vi "Untitled 1.vi"() -> ()   [LabVIEW 2015]
panel:
  in  "length":i32
  in  "x":dbl(slide) scale=0.0..10.0
  in  "y":dbl(slide) scale=0.0..10.0
  out "XY Graph":cluster{"x":dbl, "y":dbl}[](graph)
  in  "nr punktu do usuniêcia":dbl
  in  "usuñ punkt o numerze":bool
  in  "usuñ ostatni punkt":bool
  in  "rysuj punkt":bool
  in  "stop":bool
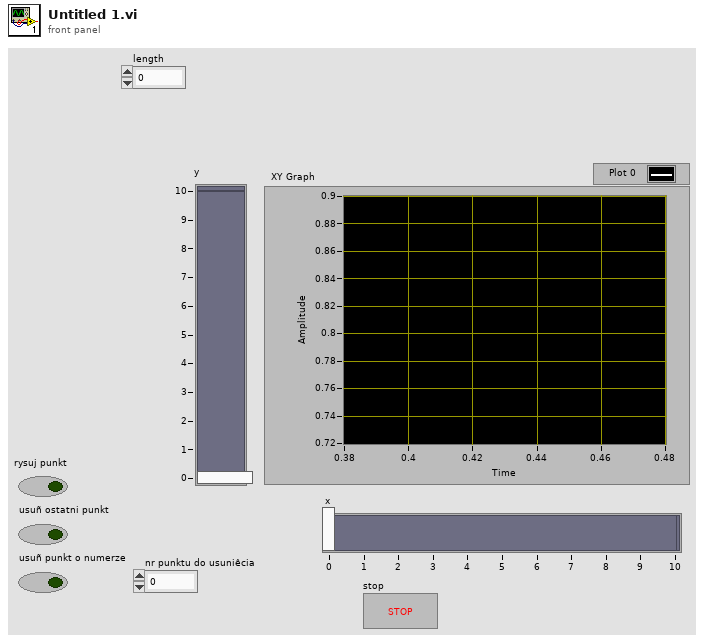
[diagram p1: front panel]
types:
  T1 = typedef "LVPoint32TypeDef.ctl" = cluster{"Horizontal":i32, "Vertical":i32}
  T2 = typedef "LVRectTypeDef.ctl" = cluster{"Left":i16, "Top":i16, "Right":i16, "Bottom":i16}
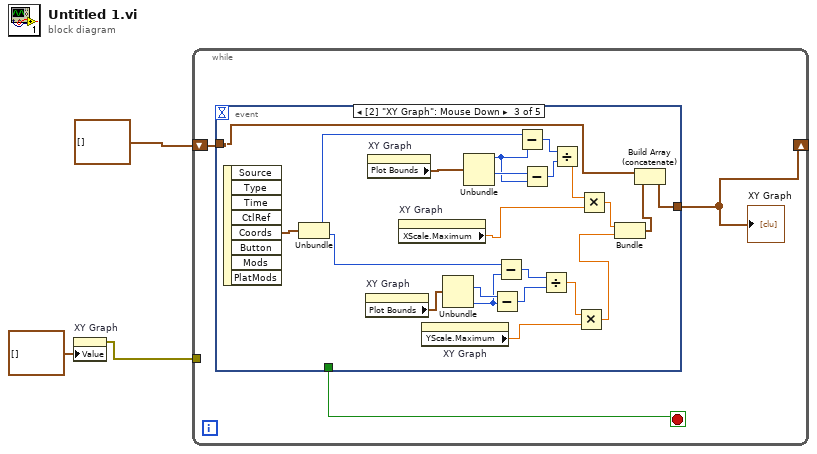
[diagram p0: block diagram]
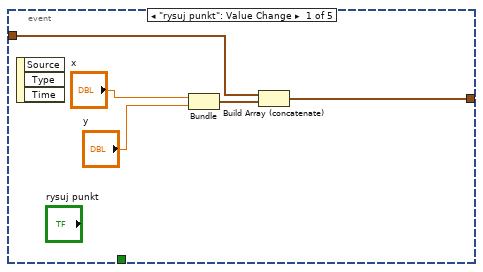
[diagram p2: hidden frame]
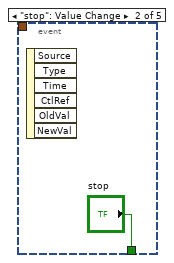
[diagram p3: hidden frame]
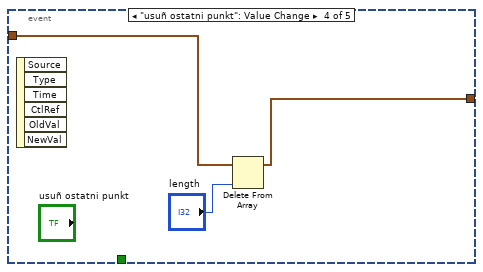
[diagram p4: hidden frame]
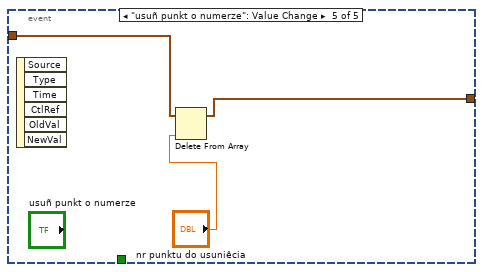
[diagram p5: hidden frame]
diagram:
  n1 = property on="XY Graph" class="XYGraph (strict)"("Value"=cluster{"x":dbl, "y":dbl}[] [] ("XY Graph")) -> (error out=w3:errorcluster)  [unwired: 2 in, 1 out]
  n2 = while {
    tunnel: w3 -> [_]
    shift-right: [w5] -> _
    shift-left: cluster{"x":dbl, "y":dbl}[] [] -> [w6]
    stop <- w4 stop-if-true
    n3 = event shown="[2] \"XY Graph\": Mouse Down" {
      selector: _ -> [_ _ _ _ _]
      dyn-events: _ -> [_ _ _ _ _]
      timeout: _ -> [_ _ _ _ _]
      tunnel: w6 -> [w11 _ w14 w37 w39]
      tunnel: [w10 _ w13 w36 w40] -> w5
      tunnel: [_ "stop" _ _ _] -> w4
      event "rysuj punkt": Value Change {
        n4 = event-data() -> ()  [unwired: 1 in, 3 out]
        n5 = Bundle("x"="x", "y"="y") -> (w7:cluster{"x":dbl, "y":dbl})  [unwired: 1 in]
        n6 = Build Array (concatenate)(w11, w7) -> (w10:cluster{"x":dbl, "y":dbl}[])
      }
      event "stop": Value Change {
        n7 = event-data() -> ()  [unwired: 1 in, 6 out]
      }
      event "XY Graph": Mouse Down {
        n8 = event-data() -> ("Coords"=w34:T1)  [unwired: 1 in, 7 out]
        n9 = Unbundle(w34) -> ("Horizontal"=w33:i32, "Vertical"=w27:i32)
        n10 = property on="XY Graph" class="XYGraph (strict)"() -> ("Plot Bounds"=w23:T2)  [unwired: 2 in, 2 out]
        n11 = property on="XY Graph" class="XYGraph (strict)"() -> ("Plot Bounds"=w32:T2)  [unwired: 2 in, 2 out]
        n12 = property on="XY Graph" class="XYGraph (strict)"() -> ("XScale.Maximum"=w26:dbl)  [unwired: 2 in, 2 out]
        n13 = property on="XY Graph" class="XYGraph (strict)"() -> ("YScale.Maximum"=w24:dbl)  [unwired: 2 in, 2 out]
        n14 = Unbundle(w23) -> ("Top"=w22:i16, "Bottom"=w19:i16)  [unwired: 2 out]
        n15 = Unbundle(w32) -> ("Left"=w18:i16, "Right"=w31:i16)  [unwired: 2 out]
        n16 = Subtract(x=w22, y=w19) -> (x-y=w21:i16)
        n17 = Subtract(x=w27, y=w19) -> (x-y=w20:i32)
        n18 = Subtract(x=w33, y=w18) -> (x-y=w30:i32)
        n19 = Subtract(x=w31, y=w18) -> (x-y=w29:i16)
        n20 = Divide(x=w20, y=w21) -> (x/y=w25:dbl)
        n21 = Divide(x=w30, y=w29) -> (x/y=w28:dbl)
        n22 = Multiply(x=w25, y=w24) -> (x*y=w16:dbl)
        n23 = Multiply(x=w28, y=w26) -> (x*y=w17:dbl)
        n24 = Bundle(w17, w16) -> (w15:cluster{dbl, dbl})  [unwired: 1 in]
        n25 = Build Array (concatenate)(w14, w15) -> (w13:cluster{"x":dbl, "y":dbl}[])
      }
      event "usuñ ostatni punkt": Value Change {
        n26 = event-data() -> ()  [unwired: 1 in, 6 out]
        n27 = Delete From Array(array=w37, index="length") -> (array with subset deleted=w36:cluster{"x":dbl, "y":dbl}[])  [unwired: 1 in, 1 out]
      }
      event "usuñ punkt o numerze": Value Change {
        n28 = event-data() -> ()  [unwired: 1 in, 6 out]
        n29 = Delete From Array(array=w39, index="nr punktu do usuniêcia") -> (array with subset deleted=w40:cluster{"x":dbl, "y":dbl}[])  [unwired: 1 in, 1 out]
      }
    }
    "XY Graph" <- w5
  }
